vi "Write Stored State DVR.vi"(8 "error in (no error)":errorcluster, 10 "Stored State DVR":refnum<data-value>, 11 "Cal Sequence Builder in":refnum<class "Cal Sequence Builder.lvclass">) -> (0 "error out":errorcluster, 3 "Cal Sequence Builder out":refnum<class "Cal Sequence Builder.lvclass">)   [LabVIEW 2015, in "Cal Sequence Builder.lvclass"]
uses:
  Cal Sequence Builder.lvclass
  State data/State Data.lvclass
  Cal Sequence Builder.lvclass/Cal Sequence Builder.ctl
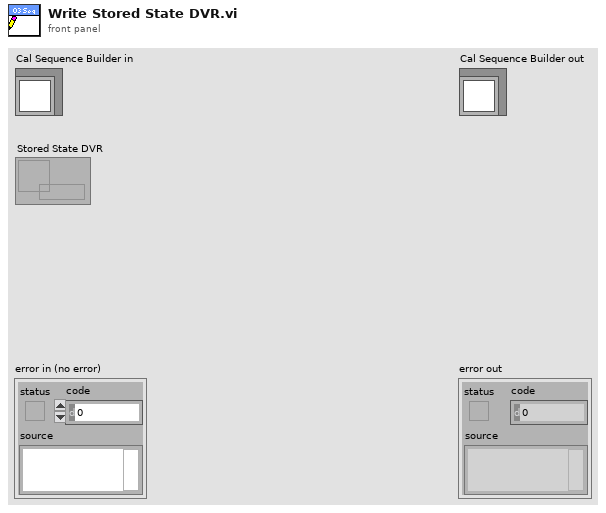
[diagram p1: front panel]
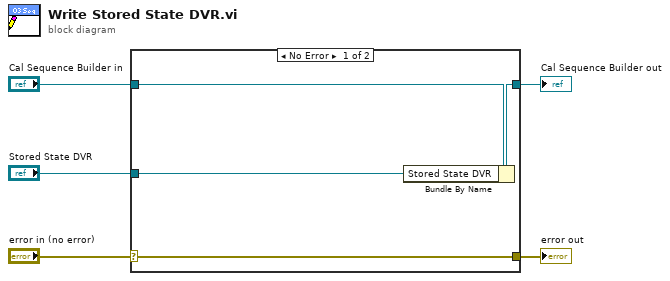
[diagram p0: block diagram]
diagram:
  n1 = case shown="No Error" "error in (no error)" {
    selector: "error in (no error)" -> [w9 w10]
    tunnel: [w9 w10] -> w4
    tunnel: [w7 w11] -> w2
    tunnel: "Cal Sequence Builder in" -> [w8 w11]
    tunnel: "Stored State DVR" -> [w6 _]
    frame No Error {
      n2 = Bundle By Name(cluster=w8, "Stored State DVR"=w6) -> (w7:refnum<class "Cal Sequence Builder.lvclass">)
    }
    frame Error {
    }
  }
  "error out" <- w4
  "Cal Sequence Builder out" <- w2
